vi "dfd_FXP PtByPt Lattice AR (basic).vi"(6 "state in":i64[](array[numeric]), 7 "FXPOPs":T5[](array[typedef]) {"source" items=["Coef a/k"=0, "Coef b/v"=7, "Input"=1, "Output"=2, "Multiplicand"=3, "Product"=4, "Sum"=5, "Delay"=6, "Gain"=8]}, 8 "filtering statistics in":T3(array[cluster]) {"statistics information"."min value" format="%.2f"; "statistics information"."max value" format="%.2f"; "Quantizer Source" items=["Coefficients a/k"=0, "Coefficients b/v"=7, "Input"=1, "Output"=2, "Multiplicand"=3, "Product"=4, "Sum"=5, "Delay"=6]}, 10 "coef k[M..1]":T4, 11 "x":T7={"value"=0, "wl"=0, "iwl"=0, "Signed"=TRUE} {"value" format="%.0x"}) -> (0 "filtering statistics out":T3(array[cluster]) {"statistics information"."min value" format="%.2f"; "statistics information"."max value" format="%.2f"; "Quantizer Source" items=["Coefficients a/k"=0, "Coefficients b/v"=7, "Input"=1, "Output"=2, "Multiplicand"=3, "Product"=4, "Sum"=5, "Delay"=6]}, 3 "filtered x":T7={"value"=0, "wl"=0, "iwl"=0, "Signed"=TRUE} {"value" format="%.0x"}, 4 "state out":i64[](array[numeric]))   [LabVIEW 2017, in "NI_DigFilter_FXP.lvlib"]
uses:
  <vilib>/addons/Digital Filter Design/NI_DigFilter_FXP.lvlib
  <vilib>/addons/Digital Filter Design/_Objects.llb/dfd_DFXP Data Type (scaler).ctl
  <vilib>/addons/Digital Filter Design/_Objects.llb/dfd_DFXP Operation Parameter.ctl
  <vilib>/addons/Digital Filter Design/_Objects.llb/dfd_Internal Quantization Srcs.ctl
  <vilib>/addons/Digital Filter Design/_Objects.llb/dfd_DFXP Data Type (vector).ctl
  <vilib>/addons/Digital Filter Design/_Objects.llb/DFD Quantization Sources.ctl
  <vilib>/addons/Digital Filter Design/_Objects.llb/DFD FXP Statistics Data.ctl
  <vilib>/addons/Digital Filter Design/NI_DigFilterLicensed.lvlib
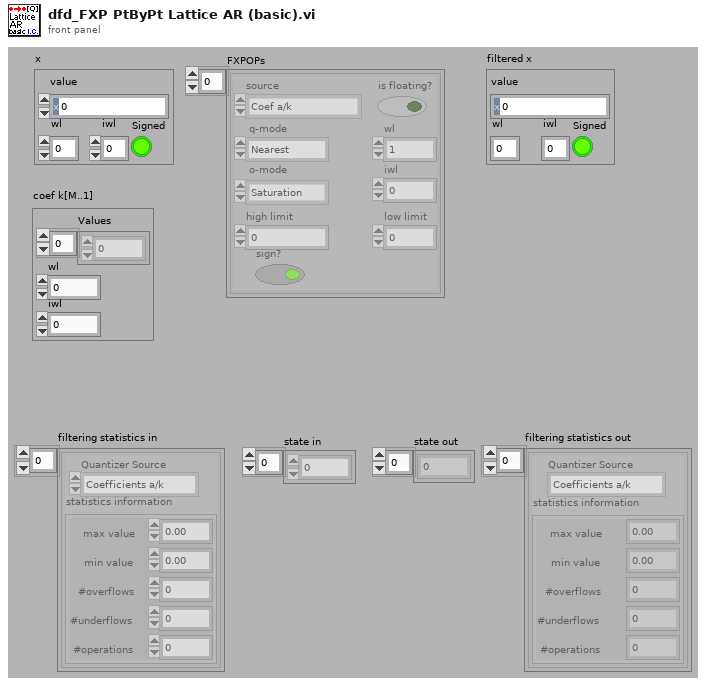
[diagram p1: front panel]
types:
  T1 = typedef "NI_DigFilterLicensed.lvlib/DFD Quantization Sources.ctl" = u16
  T2 = typedef "NI_DigFilterLicensed.lvlib/DFD FXP Statistics Data.ctl" = cluster{"max value":ext, "min value":ext, "#overflows":i32, "#underflows":i32, "#operations":i32}
  T3 = cluster{"Quantizer Source":T1, "statistics information":T2}[]
  T4 = typedef "dfd_DFXP Data Type (vector).ctl" = cluster{"Values":i64[], "wl":i16, "iwl":i16}
  T5 = typedef "dfd_DFXP Operation Parameter.ctl" = cluster{"source":T6, "is floating?":bool, "o-mode":enum16{"Saturation", "Wrap"}, "q-mode":enum16{"Nearest", "Truncation"}, "wl":i16, "high limit":i64, "low limit":i64, "iwl":i16, "sign?":bool}
  T6 = typedef "NI_DigFilterLicensed.lvlib/dfd_Internal Quantization Srcs.ctl" = u16
  T7 = typedef "dfd_DFXP Data Type (scaler).ctl" = cluster{"value":i64, "wl":i16, "iwl":i16, "Signed":bool}
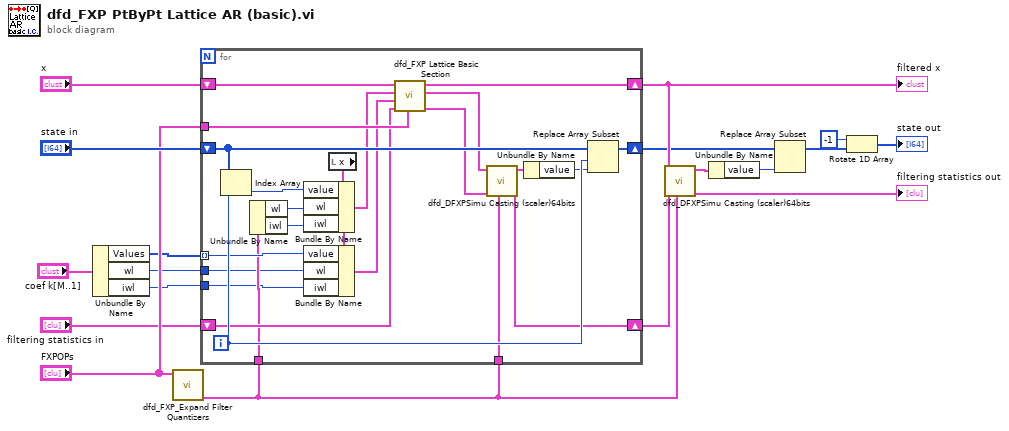
[diagram p0: block diagram]
diagram:
  n1 = Unbundle By Name("coef k[M..1]") -> ("Values"=w5:i64[], "wl"=w3:i16, "iwl"=w2:i16)
  n2 = call <vilib>:"dfd_FXP_Expand Filter Quantizers.vi"("FXPOPs"="FXPOPs") -> ("Delay"=w4:T5)  [unwired: 10 out]
  n3 = for {
    shift-right: [w33] -> w15
    shift-left: "x" -> [w36]
    shift-right: [w40] -> w13
    shift-left: "state in" -> [w41]
    tunnel: w4 -> [w29]
    tunnel: "FXPOPs" -> [w35]
    shift-right: [w30] -> w7
    shift-left: "filtering statistics in" -> [w32]
    tunnel: w5 -> [w28] mode=indexing
    tunnel: w4 -> [w24]
    tunnel: w3 -> [w21]
    tunnel: w2 -> [w20]
    i -> [w39]
    n4 = Index Array(array=w41, index=w39) -> (element=w37:i64)
    n5 = Unbundle By Name(w24) -> ("wl"=w23:i16, "iwl"=w22:i16)
    n6 = local read "x"() -> (w25:T7)
    n7 = Bundle By Name(cluster=w25, "value"=w37, "wl"=w23, "iwl"=w22) -> (w27:T7)
    n8 = Bundle By Name(cluster=w25, "value"=w28, "wl"=w21, "iwl"=w20) -> (w26:T7)
    n9 = call <vilib>:"dfd_FXP Lattice Basic Section.vi"("FXPOPs"=w35, "filtering statistics in"=w32, "k(m)"=w26, "w(m-1)"=w27, "x(m)"=w36) -> ("filtering statistics out"=w31:T3, "w(m)"=w34:T7, "x(m-1)"=w33:T7)  [unwired: 1 out]
    n10 = call <vilib>:"dfd_DFXPSimu Casting (scaler)64bits.vi"("op params"=w29, "filtering statistics in"=w31, "Value in"=w34) -> ("filtering statistics out"=w30:T3, "Value out"=w38:T7)  [unwired: 2 in, 5 out]
    n11 = Unbundle By Name(w38) -> ("value"=w19:i64)
    n12 = Replace Array Subset(array=w41, new element=w19, index=w39) -> (w40:i64[])
  }
  "filtered x" <- w15
  n13 = call <vilib>:"dfd_DFXPSimu Casting (scaler)64bits.vi"("op params"=w4, "filtering statistics in"=w7, "Value in"=w15) -> ("filtering statistics out"=→"filtering statistics out":T3, "Value out"=w11:T7)  [unwired: 2 in, 5 out]
  n14 = Unbundle By Name(w11) -> ("value"=w1:i64)
  n15 = Replace Array Subset(array=w13, new element=w1) -> (w12:i64[])  [unwired: 1 in]
  n16 = Rotate 1D Array(1:w12, 2:-1 ("n")) -> (0:→"state out":i64[])
